vi "Ctor.vi"(8 "error in (no error)":errorcluster, 10 "Database":refnum<class "Database Platform.lvclass">) -> (0 "error out":errorcluster, 3 "Entity Manager out":refnum<class "Entity Manager.lvclass">)   [LabVIEW 2020, in "Conditu2.lvlib" / "Entity Manager.lvclass"]
uses:
  Entity Manager.lvclass
  Database Platform/Database Platform.lvclass
  Entity Manager.lvclass/Entity Manager.ctl
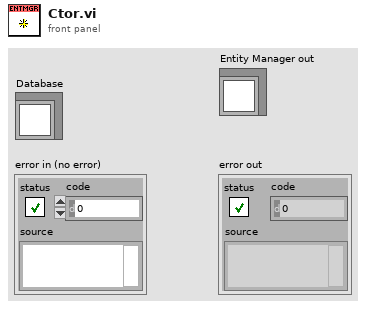
[diagram p1: front panel]
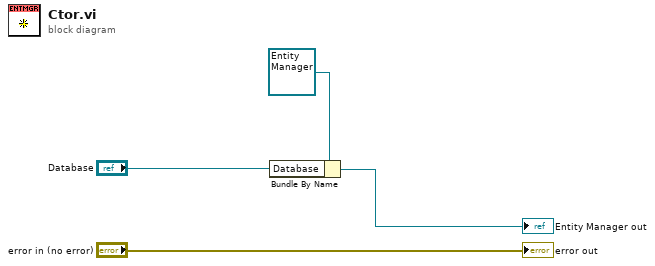
[diagram p0: block diagram]
diagram:
  n1 = Bundle By Name(cluster=refnum<class "Entity Manager.lvclass"> refnum ("Entity Manager in"), "Database"="Database") -> (→"Entity Manager out":refnum<class "Entity Manager.lvclass">)
  "error out" <- "error in (no error)"
